vi "reverse.vi"(8 "Error in":errorcluster caption="Error in (no error)", 11 "Reverse Parameters (in)":T1) -> (0 "Error out":errorcluster, 3 "Reverse Parameters (out)":T1, 4 "Reverse Time (ms)":dbl)   [LabVIEW 2018]
uses:
  Controls/reverse_parameters.ctl
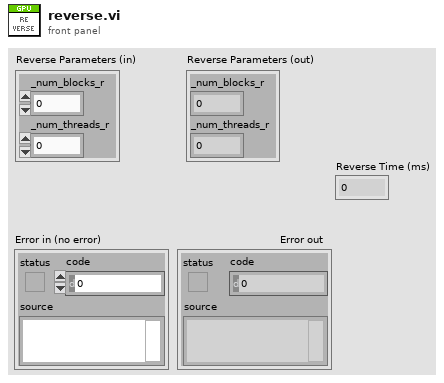
[diagram p1: front panel]
types:
  T1 = typedef "reverse_parameters.ctl" = cluster{"_num_blocks_r":i32, "_num_threads_r":i32}
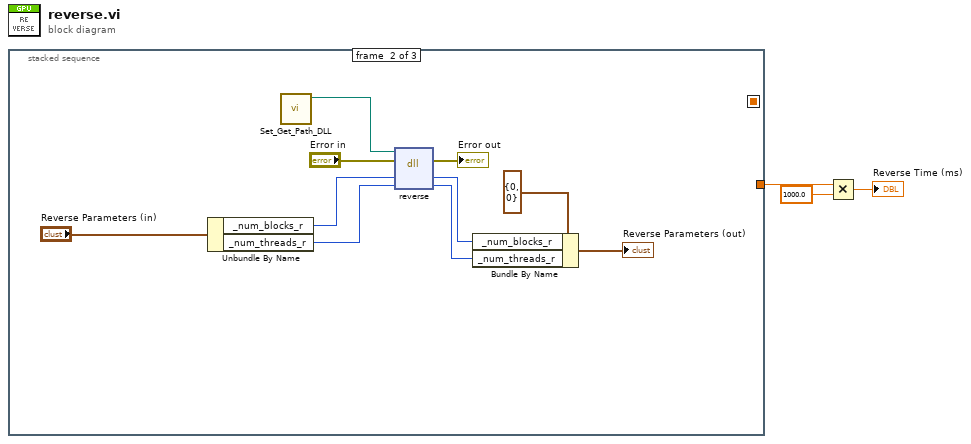
[diagram p0: block diagram]
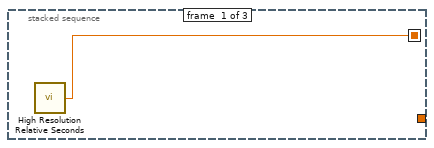
[diagram p2: hidden frame]
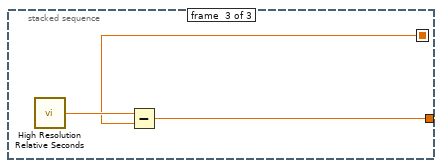
[diagram p3: hidden frame]
diagram:
  n1 = stacked-sequence {
    seq-local: [w4 _ _] -> [_ _ w16]
    tunnel: [_ _ w15] -> w1
    frame #0 {
      n2 = call <vilib>:"High Resolution Relative Seconds.vi"() -> ("relative seconds"=w4:dbl)
    }
    frame #1 {
      n3 = Unbundle By Name("Reverse Parameters (in)") -> ("_num_blocks_r"=w12:i32, "_num_threads_r"=w11:i32)
      n4 = call "Set_Get_Path_DLL.vi"() -> ("path DLL Out"=w5:path)  [unwired: 11 in]
      n5 = dll-call lib="C:/Users/AUTIS/Documents/TFG/Proyecto/Visual Studio/SR_GPU_TOOLKIT_INIT/x64/Release/SR_GPU_TOOLKIT.dll" fn="reverse"(path in=w5, error in="Error in", "_num_blocks_th"=w12, "_num_threads_th"=w11) -> (error out=→"Error out":errorcluster, "_num_blocks_th"=w10:i32, "_num_threads_th"=w9:i32)  [unwired: 2 in, 1 out]
      n6 = Bundle By Name(cluster=T1 {"_num_blocks_r"=0, "_num_threads_r"=0} ("Reverse Parameters 2"), "_num_blocks_r"=w10, "_num_threads_r"=w9) -> (→"Reverse Parameters (out)":T1)
    }
    frame #2 {
      n7 = call <vilib>:"High Resolution Relative Seconds.vi"() -> ("relative seconds"=w17:dbl)
      n8 = Subtract(x=w17, y=w16) -> (x-y=w15:dbl)
    }
  }
  n9 = Multiply(x=w1, y=1000.0) -> (x*y=→"Reverse Time (ms)":dbl)
